vi "Generator Lesson 3.vi"() -> ()   [LabVIEW 2024]
uses:
  <vilib>/Instr/_visa.llb/VISA Configure Serial Port (Instr).vi
panel:
  in  "Motor Speed":dbl(slide) scale=0.0..255.0
  in  "stop":bool
  out "Waveform Chart":dbl(graph)
  in  "VISA resource name":refnum<visa-resource-name>
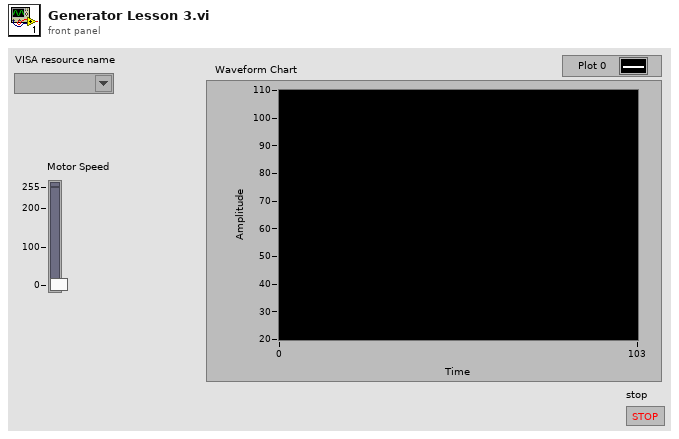
[diagram p1: front panel]
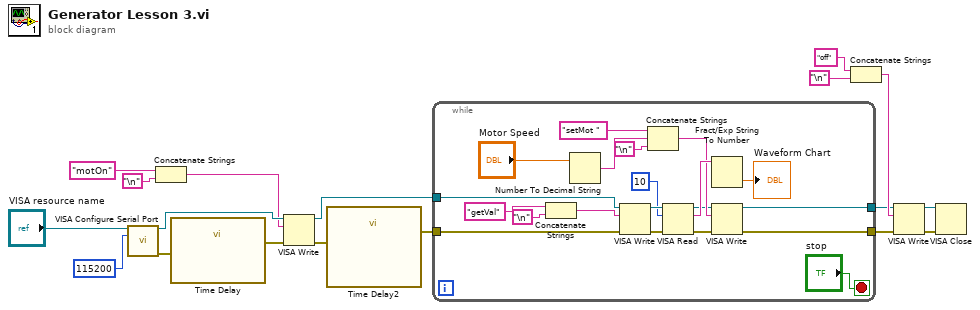
[diagram p0: block diagram]
diagram:
  n1 = call-poly "VISA Configure Serial Port"("VISA resource name"="VISA resource name", "baud rate (9600)"=u32 115200) -> ("VISA resource name out"=w15:refnum<visa-resource-name>, "error out"=w16:errorcluster)  [unwired: 12 in]
  n2 = Concatenate Strings("motOn", "\n") -> (w11:string)
  n3 = call "Time Delay"("error in (no error)"=w16) -> ("error out"=w14:errorcluster)  [unwired: 10 in]
  n4 = VISA Write(VISA resource name=w15, write buffer=w11, error in (no error)=w14) -> (VISA resource name out=w8:refnum<visa-resource-name>, error out=w10:errorcluster)  [unwired: 1 out]
  n5 = call "Time Delay2"("error in (no error)"=w10) -> ("error out"=w9:errorcluster)  [unwired: 10 in]
  n6 = while {
    tunnel: w9 -> [w36]
    tunnel: w8 -> [w35]
    tunnel: [w20] -> w4
    tunnel: [w19] -> w3
    stop <- "stop" stop-if-true
    n7 = Concatenate Strings("getVal", "\n") -> (w34:string)
    n8 = Number To Decimal String(number="Motor Speed") -> (decimal integer string=w21:string)  [unwired: 1 in]
    n9 = VISA Write(VISA resource name=w35, write buffer=w34, error in (no error)=w36) -> (VISA resource name out=w33:refnum<visa-resource-name>, error out=w32:errorcluster)  [unwired: 1 out]
    n10 = Concatenate Strings("setMot ", w21, "\n") -> (w25:string)
    n11 = VISA Read(VISA resource name=w33, byte count=u32 10, error in (no error)=w32) -> (VISA resource name out=w24:refnum<visa-resource-name>, read buffer=w30:string, error out=w23:errorcluster)  [unwired: 1 out]
    n12 = Fract/Exp String To Number(string=w30) -> (number=→"Waveform Chart":dbl)  [unwired: 3 in, 1 out]
    n13 = VISA Write(VISA resource name=w24, write buffer=w25, error in (no error)=w23) -> (VISA resource name out=w20:refnum<visa-resource-name>, error out=w19:errorcluster)  [unwired: 1 out]
  }
  n14 = Concatenate Strings("off", "\n") -> (w5:string)
  n15 = VISA Write(VISA resource name=w4, write buffer=w5, error in (no error)=w3) -> (VISA resource name out=w2:refnum<visa-resource-name>, error out=w1:errorcluster)  [unwired: 1 out]
  n16 = VISA Close(VISA resource name=w2, error in (no error)=w1) -> ()  [unwired: 1 out]
